vi "Write Results in Filename.vi"(8 "error in (no error)":errorcluster, 10 "Results in Filename":bool, 11 "POLARIS TA Focus Display in":refnum<class "POLARIS TA Focus Display.lvclass">) -> (0 "error out":errorcluster, 3 "POLARIS TA Focus Display out":refnum<class "POLARIS TA Focus Display.lvclass">)   [LabVIEW 2014, in "POLARIS TA Focus Display.lvlib" / "POLARIS TA Focus Display.lvclass"]
uses:
  POLARIS TA Focus Display.lvclass
  POLARIS TA Focus Display.lvclass/POLARIS TA Focus Display.ctl
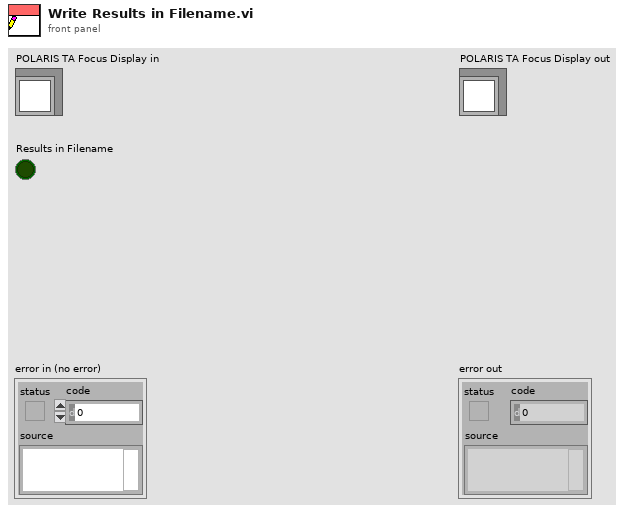
[diagram p1: front panel]
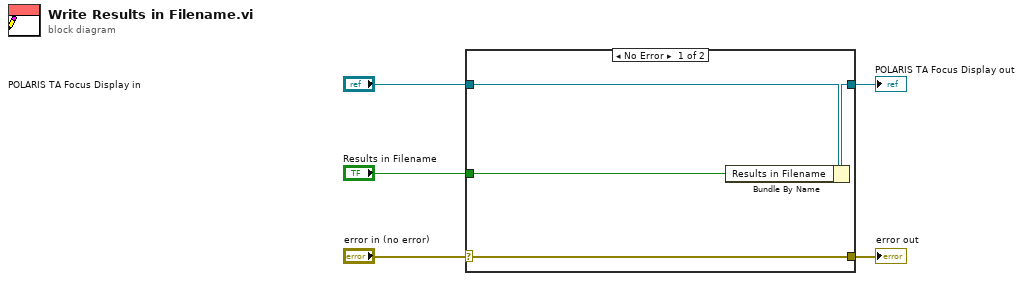
[diagram p0: block diagram]
diagram:
  n1 = case shown="No Error" "error in (no error)" {
    selector: "error in (no error)" -> [w9 w10]
    tunnel: [w9 w10] -> w4
    tunnel: [w7 w11] -> w2
    tunnel: "POLARIS TA Focus Display in" -> [w8 w11]
    tunnel: "Results in Filename" -> [w6 _]
    frame No Error {
      n2 = Bundle By Name(cluster=w8, "Results in Filename"=w6) -> (w7:refnum<class "POLARIS TA Focus Display.lvclass">)
    }
    frame Error {
    }
  }
  "error out" <- w4
  "POLARIS TA Focus Display out" <- w2
